vi "IDtoNode.vi"(8 "error in":errorcluster, 11 "ID":string) -> (0 "error out":errorcluster, 2 "invalid Id":bool, 3 "node ref":T1)   [LabVIEW 2013, in "NISE_CEF_Node.lvclass"]
doc: "This VI obtains the reference to a node from its ID."
uses:
  NISE_CEF_Node.lvclass
  NodeRef.ctl
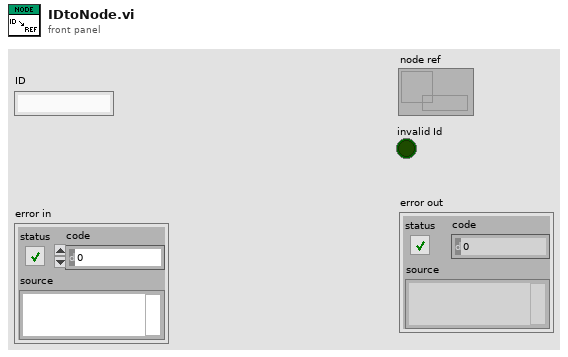
[diagram p1: front panel]
types:
  T1 = typedef "NISE_CEF_Node.lvclass/NodeRef.ctl" = refnum<data-value>
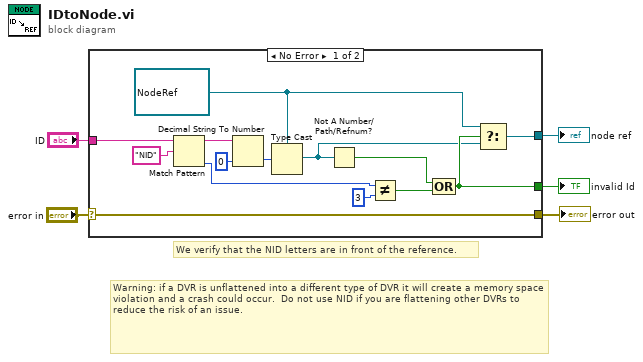
[diagram p0: block diagram]
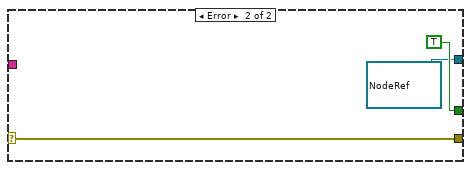
[diagram p2: hidden frame]
diagram:
  # "Warning: if a DVR is unflattened into a different type of DVR it will create a memory space violation and a crash could occur.  Do not use NID if you are flattening other DVRs to reduce the risk of an issue."
  # "We verify that the NID letters are in front of the reference."
  n1 = case shown="No Error" "error in" {
    selector: "error in" -> [w6 w22]
    tunnel: [w19 T1 refnum ("root")] -> w5
    tunnel: "ID" -> [w13 _]
    tunnel: [w6 w22] -> w2
    tunnel: [w12 TRUE] -> w1
    frame No Error {
      w10 = T1 refnum ("root")
      n2 = Match Pattern(string=w13, regular expression="NID") -> (after substring=w9:string, offset past match=w17:i32)  [unwired: 1 in, 2 out]
      n3 = Decimal String To Number(string=w9, default (0L)=u32 0) -> (number=w7:u32)  [unwired: 1 in, 1 out]
      n4 = Type Cast(type=w10, x=w7) -> (*(type *) &x=w11:T1)
      n5 = Not A Number/Path/Refnum?(number/path/refnum=w11) -> (NaN/Path/Refnum?=w14:bool)
      n6 = Not Equal?(x=w17, y=3) -> (x != y?=w15:bool)
      n7 = Compound Arithmetic op=OR(w14, w15) -> (w12:bool)
      n8 = Select(t=w10, s=w12, f=w11) -> (s? t:f=w19:T1)
    }
    frame Error {
    }
  }
  "node ref" <- w5
  "error out" <- w2
  "invalid Id" <- w1
